vi "GetImages.vi"(4 "File type":T1, 5 "Disabled":bool, 6 "Background Color":u32(colorbox), 7 "image directory":path, 8 "error in":errorcluster, 11 "Path in":refnum<class "Path.lvclass">) -> (0 "error out":errorcluster, 3 "Path out":refnum<class "Path.lvclass">)   [LabVIEW 2014, in "Path.lvclass"]
uses:
  Path.lvclass
  Control/ImageTypes.ctl
  Path.lvclass/Path.ctl
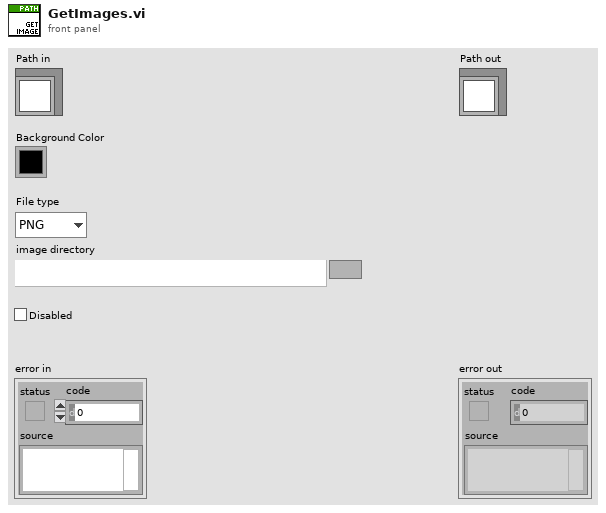
[diagram p1: front panel]
types:
  T1 = typedef "ImageTypes.ctl" = enum16{"PNG", "JPEG", "BMP"}
  T2 = typedef "LVRectTypeDef.ctl" = cluster{"Left":i16, "Top":i16, "Right":i16, "Bottom":i16}
  T3 = typedef "imagedata.ctl" = cluster{"image type":i32, "image depth":i32, "image":u8[], "mask":u8[], "colors":u32[], "Rectangle":cluster{"left":i16, "top":i16, "right":i16, "bottom":i16}}
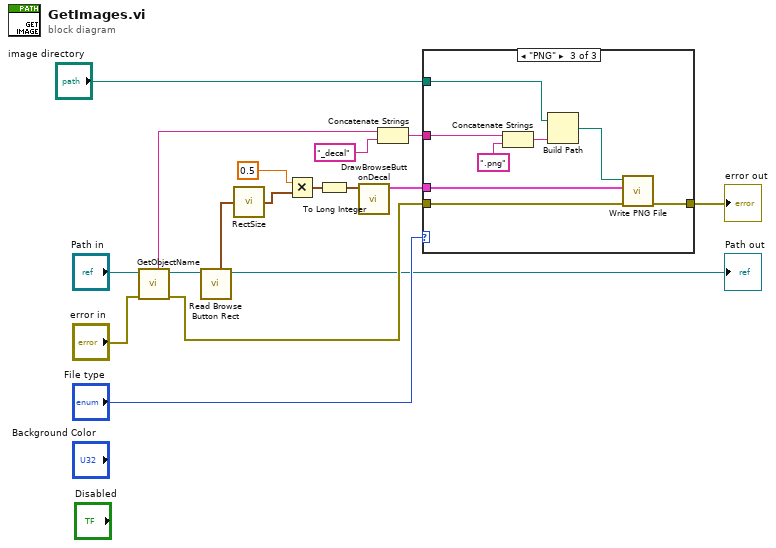
[diagram p0: block diagram]
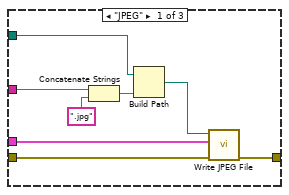
[diagram p2: hidden frame]
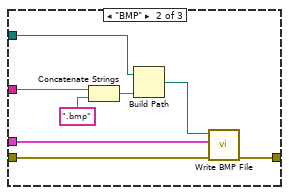
[diagram p3: hidden frame]
diagram:
  n1 = call-dynamic "GetObjectName.vi"("error in"="error in", "GObject in"="Path in") -> ("error out"=w4:errorcluster, "GObject out"=w9:refnum<class "Path.lvclass">, "Name"=w6:string)  [unwired: 5 in]
  n2 = call "Read Browse Button Rect.vi"("Path in"=w9) -> ("Path out"=→"Path out":refnum<class "Path.lvclass">, "Browse Button Rect"=w17:T2)  [unwired: 7 in]
  n3 = call <vilib>:"RectSize.vi"("rect"=w17) -> ("point"=w16:cluster{"x":i16, "y":i16})
  n4 = Multiply(x=0.5, y=w16) -> (x*y=w14:cluster{"x":dbl, "y":dbl})
  n5 = To Long Integer(number=w14) -> (32bit integer=w13:cluster{"x":i32, "y":i32})
  n6 = call "DrawBrowseButtonDecal.vi"("Size"=w13) -> ("image"=w11:T3)  [unwired: 10 in]
  n7 = Concatenate Strings(w6, "_decal" ("string")) -> (w7:string)
  n8 = case shown="\"PNG\"" "File type" {
    tunnel: w11 -> [w25 w33 w41]
    tunnel: [w24 w32 w40] -> w3
    tunnel: w4 -> [w23 w31 w39]
    tunnel: w7 -> [w22 w30 w38]
    tunnel: "image directory" -> [w18 w26 w34]
    frame "JPEG" {
      n9 = Concatenate Strings(w22, ".jpg" ("string")) -> (w20:string)
      n10 = Build Path(base path=w18, name or relative path=w20) -> (appended path=w19:path)
      n11 = call <vilib>:"Write JPEG File.vi"("error in (no error)"=w23, "image data"=w25, "path to JPEG file"=w19) -> ("error out"=w24:errorcluster)  [unwired: 7 in, 1 out]
    }
    frame "BMP" {
      n12 = Concatenate Strings(w30, ".bmp" ("string")) -> (w28:string)
      n13 = Build Path(base path=w26, name or relative path=w28) -> (appended path=w27:path)
      n14 = call <vilib>:"Write BMP File.vi"("error in (no error)"=w31, "image data"=w33, "path to BMP file"=w27) -> ("error out"=w32:errorcluster)  [unwired: 7 in, 1 out]
    }
    frame "PNG" {
      n15 = Concatenate Strings(w38, ".png" ("string")) -> (w36:string)
      n16 = Build Path(base path=w34, name or relative path=w36) -> (appended path=w35:path)
      n17 = call <vilib>:"Write PNG File.vi"("error in (no error)"=w39, "image data"=w41, "path to PNG file"=w35) -> ("error out"=w40:errorcluster)  [unwired: 7 in, 1 out]
    }
  }
  "error out" <- w3
